vi "PID.vi"(0 "setpoint":dbl step=0.01 format="%.2f", 1 "X1(SetState)":T1(ring)=enum."max", 2 "reinitialize? (F)":bool, 5 "process variable":dbl step=0.01 format="%.2f", 7 "PID param":T2={"proportional gain (Kc)"=1.0, "integral time (Ti, s)"=10.0, "derivative time (Td, s)"=1.0, "output high"=100.0, "alr value"=0.0, "output low"=0.0, "output rate (EGU/s)"=1.0, "dt (s)"=-1.0} {"dt (s)" format="%.3f"; "output rate (EGU/s)" format="%.2f"; "output low" format="%.2f"; "alr value" format="%.2f"; "output high" format="%.2f"; "derivative time (Td, s)" format="%.3f"; "integral time (Ti, s)" format="%.3f"; "proportional gain (Kc)" format="%.3f"}, 9 "manual control":dbl format="%.2f") -> (4 "set output":dbl format="%.2f", 6 "output":dbl format="%.2f", 10 "dt out (s)":dbl format="%.3f")   [LabVIEW 2019, in "control.lvlib"]
uses:
  control.lvlib
  ctl/PID param.ctl
panel:
  # "Входы\nX1(SetState) заданное состояние\n     0 – аварийное значение\n     1 – минимум\n     2 – стоп\n     3 – ручной\n     4 – автомат\n     5 – максимум"
  # "PID gains"
  # "output param"
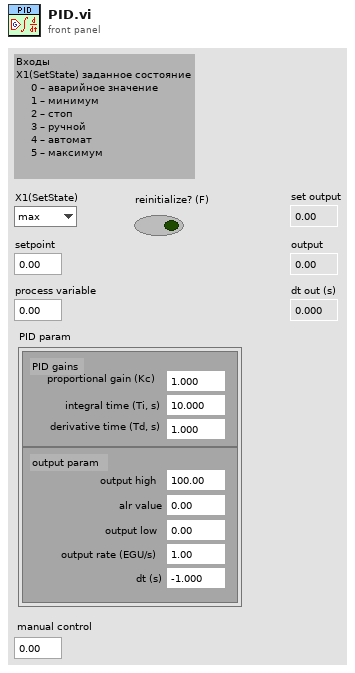
[diagram p1: front panel]
types:
  T1 = enum8{"alarm", "min", "stop", "hand", "auto", "max"}
  T2 = typedef "control.lvlib/PID param.ctl" = cluster{"proportional gain (Kc)":dbl, "integral time (Ti, s)":dbl, "derivative time (Td, s)":dbl, "output high":dbl, "alr value":dbl, "output low":dbl, "output rate (EGU/s)":dbl, "dt (s)":dbl}
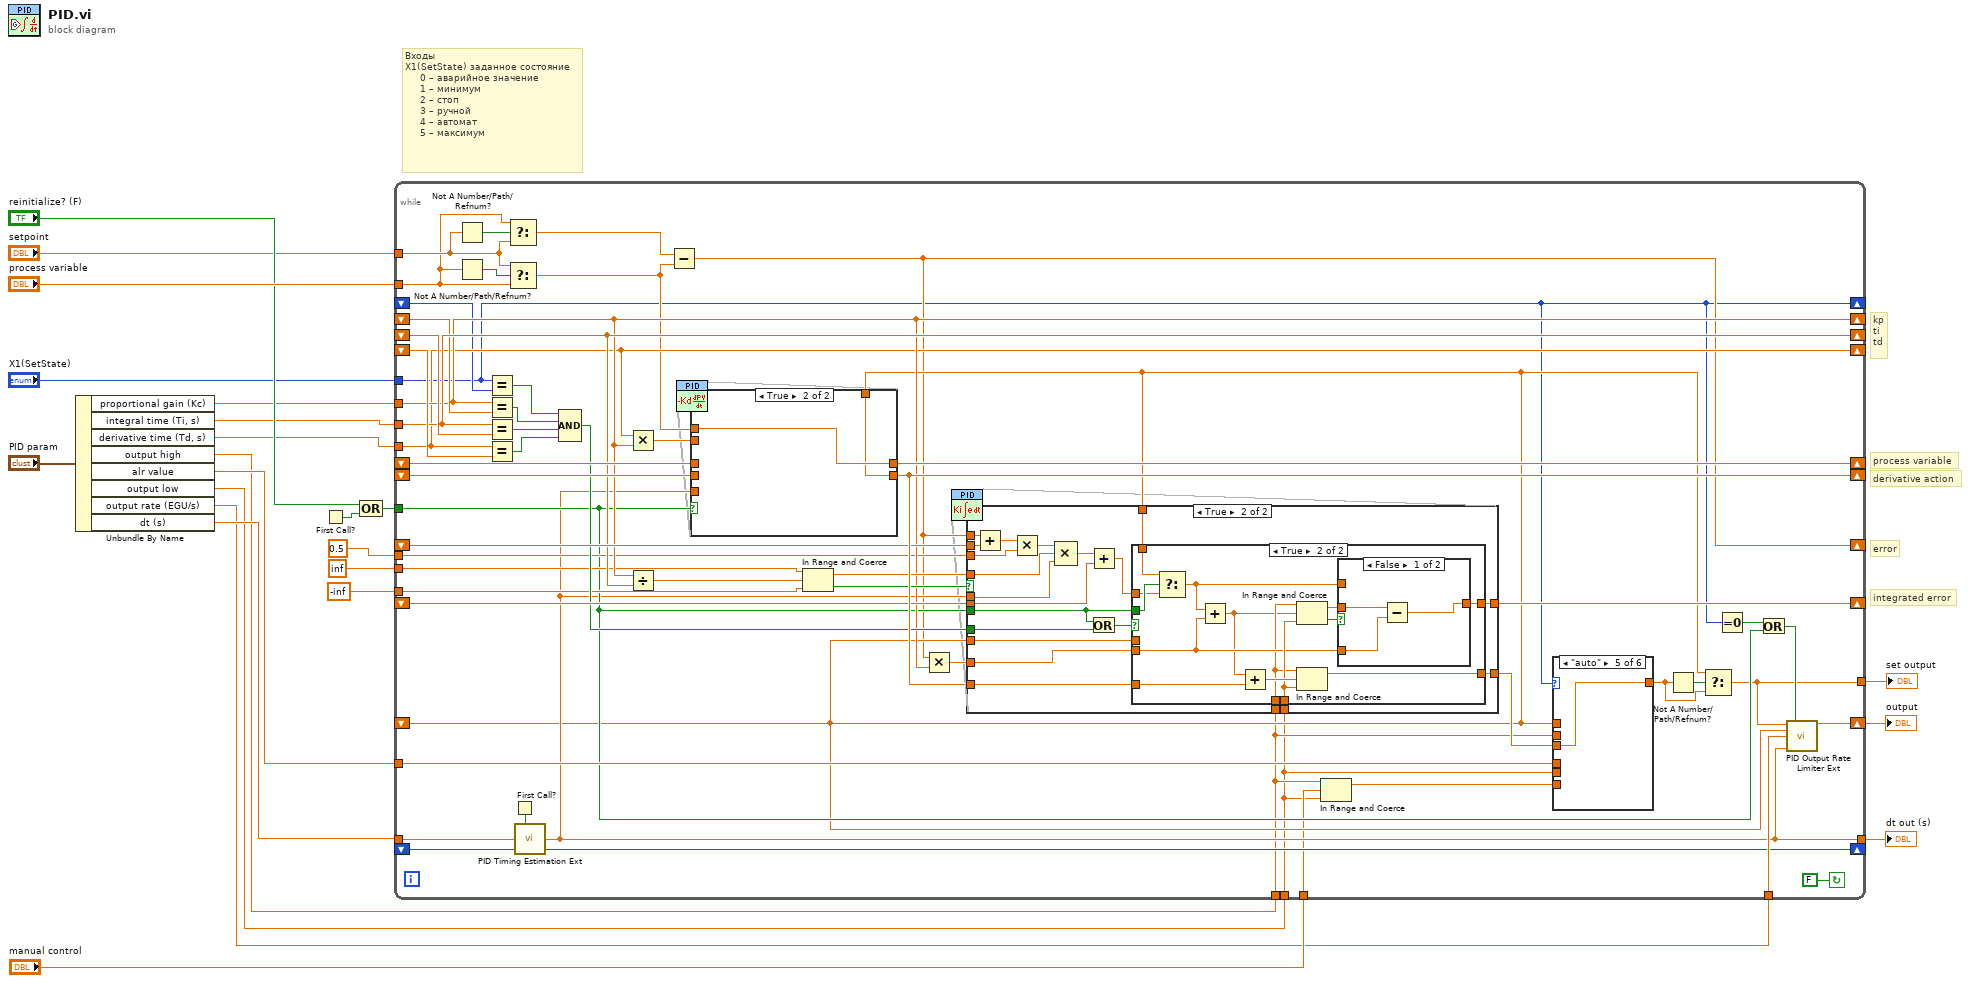
[diagram p0: block diagram]
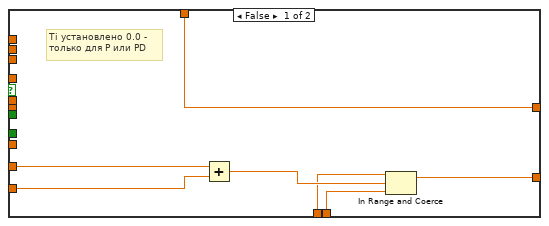
[diagram p2: hidden frame]
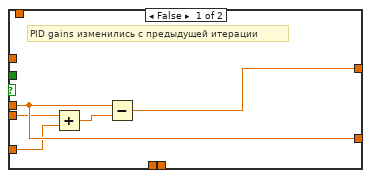
[diagram p3: hidden frame]
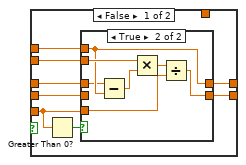
[diagram p5: hidden frame]
diagram:
  # "derivative action"
  # "process variable"
  # "kp\nti\ntd"
  # "error"
  # "integrated error"
  # "Входы\nX1(SetState) заданное состояние\n     0 – аварийное значение\n     1 – минимум\n     2 – стоп\n     3 – ручной\n     4 – автомат\n     5 – максимум"
  n1 = Unbundle By Name("PID param") -> ("proportional gain (Kc)"=w13:dbl, "integral time (Ti, s)"=w14:dbl, "derivative time (Td, s)"=w15:dbl, "output high"=w5:dbl, "alr value"=w7:dbl, "output low"=w4:dbl, "output rate (EGU/s)"=w3:dbl, "dt (s)"=w6:dbl)
  n2 = First Call?() -> (First Call?: T/F=w22:bool)
  n3 = Compound Arithmetic op=OR("reinitialize? (F)", w22) -> (w12:bool)
  n4 = while {
    tunnel: w12 -> [w37]
    shift-right: [w58] -> _
    shift-left: _ -> [w59]
    shift-right: [w60] -> _
    shift-left: _ -> [w77]
    shift-right: [w53] -> _
    shift-left: _ -> [w78]
    tunnel: w13 -> [w58]
    tunnel: w14 -> [w60]
    tunnel: w15 -> [w53]
    tunnel: w6 -> [w52]
    tunnel: w5 -> [w29]
    tunnel: w4 -> [w28]
    tunnel: "process variable" -> [w40]
    shift-right: [w73] -> _
    shift-left: _ -> [w72]
    shift-right: [w71] -> _
    shift-left: _ -> [w65]
    shift-right: [w26] -> _
    shift-left: _ -> [w70]
    shift-right: [w69] -> _
    shift-left: _ -> [w68]
    tunnel: 0.5 ("y") -> [w57]
    tunnel: inf ("upper limit") -> [w55]
    tunnel: -inf ("lower limit") -> [w56]
    tunnel: [w34] -> w11
    tunnel: "manual control" -> [w30]
    tunnel: w3 -> [w35]
    shift-right: [w38] -> w9
    shift-left: _ -> [w33]
    tunnel: w7 -> [w48]
    tunnel: "X1(SetState)" -> [w25]
    shift-right: [w25] -> _
    shift-left: _ -> [w47]
    tunnel: "setpoint" -> [w42]
    shift-right: [w32] -> _
    shift-left: _ -> [w31]
    tunnel: [w23] -> w1
    stop <- FALSE continue-if-true
    n5 = Not A Number/Path/Refnum?(number/path/refnum=w42) -> (NaN/Path/Refnum?=w43:bool)
    n6 = Not A Number/Path/Refnum?(number/path/refnum=w40) -> (NaN/Path/Refnum?=w44:bool)
    n7 = Equal?(x=w25, y=w47) -> (x = y?=w46:bool)
    n8 = Equal?(x=w58, y=w59) -> (x = y?=w75:bool)
    n9 = Equal?(x=w60, y=w77) -> (x = y?=w74:bool)
    n10 = Equal?(x=w53, y=w78) -> (x = y?=w76:bool)
    n11 = Select(t=w40, s=w43, f=w42) -> (s? t:f=w41:dbl)
    n12 = Select(t=w42, s=w44, f=w40) -> (s? t:f=w45:dbl)
    n13 = First Call?() -> (First Call?: T/F=w24:bool)
    n14 = call "PID Timing Estimation Ext.vi"("R"=w24, "dt (s) in"=w52, "Tick old"=w31) -> ("dt (s) out"=w34:dbl, "Tick"=w32:u32)  [unwired: 5 in]
    n15 = Compound Arithmetic op=AND(w46, w75, w74, w76) -> (w61:bool)
    n16 = Multiply(x=w53, y=w58) -> (x*y=w64:dbl)
    n17 = Divide(x=w58, y=w60) -> (x/y=w63:dbl)
    n18 = Subtract(x=w41, y=w45) -> (x-y=w26:dbl)
    n19 = case shown="True" w37 {
      tunnel: w72 -> [w137 _]
      tunnel: w64 -> [w134 _]
      tunnel: w45 -> [w136 w148]
      tunnel: [w133 w148] -> w73
      tunnel: [w135 w147] -> w71
      tunnel: w65 -> [w131 _]
      tunnel: w34 -> [w130 _]
      tunnel: w33 -> [_ w147]
      frame False {
        n20 = Greater Than 0?(x=w130) -> (x > 0?=w132:bool)
        n21 = case shown="True" w132 {
          tunnel: w137 -> [w139 w140]
          tunnel: w130 -> [_ w145]
          tunnel: w136 -> [_ w141]
          tunnel: [w138 w144] -> w135
          tunnel: w134 -> [_ w143]
          tunnel: [w139 w141] -> w133
          tunnel: w131 -> [w138 _]
          frame False {
            # "dt = 0 min"
          }
          frame True {
            n22 = Subtract(x=w140, y=w141) -> (x-y=w142:dbl)
            n23 = Multiply(x=w143, y=w142) -> (x*y=w146:dbl)
            n24 = Divide(x=w146, y=w145) -> (x/y=w144:dbl)
          }
        }
      }
      frame True {
      }
    }
    n25 = In Range and Coerce(upper limit=w55, x=w63, lower limit=w56) -> (coerced(x)=w67:dbl, In Range?=w66:bool)
    n26 = Multiply(x=w26, y=w58) -> (x*y=w62:dbl)
    n27 = case shown="True" w66 {
      tunnel: w26 -> [_ w105]
      tunnel: w70 -> [_ w106]
      tunnel: w68 -> [_ w101]
      tunnel: [w79 w96] -> w69
      tunnel: w67 -> [_ w94]
      tunnel: w62 -> [w84 w99]
      tunnel: [w85 w95] -> w50
      tunnel: w33 -> [_ w97]
      tunnel: w71 -> [w83 w93]
      tunnel: w37 -> [_ w92]
      tunnel: w61 -> [_ w91]
      tunnel: w34 -> [_ w90]
      tunnel: w29 -> [w81 w88]
      tunnel: w28 -> [w80 w89]
      tunnel: w57 -> [_ w87]
      tunnel: w33 -> [w79 w86]
      frame False {
        # "Ti установлено 0.0 -\nтолько для P или PD"
        n28 = Add(x=w84, y=w83) -> (x+y=w82:dbl)
        n29 = In Range and Coerce(upper limit=w81, x=w82, lower limit=w80) -> (coerced(x)=w85:dbl)  [unwired: 1 out]
      }
      frame True {
        n30 = Add(x=w105, y=w106) -> (x+y=w104:dbl)
        n31 = Multiply(x=w104, y=w87) -> (x*y=w103:dbl)
        n32 = Compound Arithmetic op=MULTIPLY(w103, w94, w90) -> (w102:dbl)
        n33 = Add(x=w102, y=w101) -> (x+y=w100:dbl)
        n34 = Or(x=w92, y=w91) -> (x .or. y?=w98:bool)
        n35 = case shown="True" w98 {
          tunnel: w100 -> [_ w112]
          tunnel: w99 -> [w109 w118]
          tunnel: w97 -> [w111 _]
          tunnel: w92 -> [_ w115]
          tunnel: [w110 w120] -> w96
          tunnel: [w111 w124] -> w95
          tunnel: w93 -> [w108 w123]
          tunnel: w89 -> [_ w122]
          tunnel: w88 -> [_ w117]
          tunnel: w86 -> [_ w114]
          frame False {
            # "PID gains изменились с предыдущей итерации"
            n36 = Add(x=w109, y=w108) -> (x+y=w107:dbl)
            n37 = Subtract(x=w111, y=w107) -> (x-y=w110:dbl)
          }
          frame True {
            n38 = Select(t=w114, s=w115, f=w112) -> (s? t:f=w113:dbl)
            n39 = Add(x=w113, y=w118) -> (x+y=w116:dbl)
            n40 = Add(x=w116, y=w123) -> (x+y=w125:dbl)
            n41 = In Range and Coerce(upper limit=w117, x=w116, lower limit=w122) -> (coerced(x)=w119:dbl, In Range?=w121:bool)
            n42 = In Range and Coerce(upper limit=w117, x=w125, lower limit=w122) -> (coerced(x)=w124:dbl)  [unwired: 1 out]
            n43 = case shown="False" w121 {
              tunnel: w113 -> [_ w129]
              tunnel: [w126 w129] -> w120
              tunnel: w119 -> [w128 _]
              tunnel: w118 -> [w127 _]
              frame False {
                n44 = Subtract(x=w128, y=w127) -> (x-y=w126:dbl)
              }
              frame True {
              }
            }
          }
        }
      }
    }
    n45 = In Range and Coerce(upper limit=w29, x=w30, lower limit=w28) -> (coerced(x)=w27:dbl)  [unwired: 1 out]
    n46 = case shown="\"auto\"" w25 {
      tunnel: w33 -> [_ _ w151 _ _ _]
      tunnel: w50 -> [_ _ _ _ w153 _]
      tunnel: w27 -> [_ _ _ w152 _ _]
      tunnel: [w149 w150 w151 w152 w153 w154] -> w49
      tunnel: w48 -> [w149 _ _ _ _ _]
      tunnel: w29 -> [_ _ _ _ _ w154]
      tunnel: w28 -> [_ w150 _ _ _ _]
      frame "alarm", Default {
      }
      frame "min" {
      }
      frame "stop" {
      }
      frame "hand" {
      }
      frame "auto" {
      }
      frame "max" {
      }
    }
    n47 = Not A Number/Path/Refnum?(number/path/refnum=w49) -> (NaN/Path/Refnum?=w51:bool)
    n48 = Select(t=w33, s=w51, f=w49) -> (s? t:f=w23:dbl)
    n49 = Equal To 0?(x=w25) -> (x = 0?=w39:bool)
    n50 = Or(x=w39, y=w37) -> (x .or. y?=w36:bool)
    n51 = call "PID Output Rate Limiter Ext.vi"("input (controller output)"=w23, "reinitialize? (F)"=w36, "output old"=w33, "output rate (EGU/s)"=w35, "dt (s)"=w34) -> ("output"=w38:dbl)  [unwired: 8 in, 2 out]
  }
  "output" <- w9
  "dt out (s)" <- w11
  "set output" <- w1
